vi "addNewMeasuredTemperature.vi"(8 "error in (no error)":errorcluster, 10 "Temperature Measured":dbl[unit]=275.15 min=271.15 max=275.15 format="%.1f", 11 "TestMonitor in":refnum<class "TestMonitor.lvclass">) -> (0 "error out":errorcluster, 3 "TestMonitor out":refnum<class "TestMonitor.lvclass">)   [LabVIEW 2013, in "TestMonitor.lvclass"]
uses:
  TestMonitor.lvclass
  TestMonitor.lvclass/TestMonitor.ctl
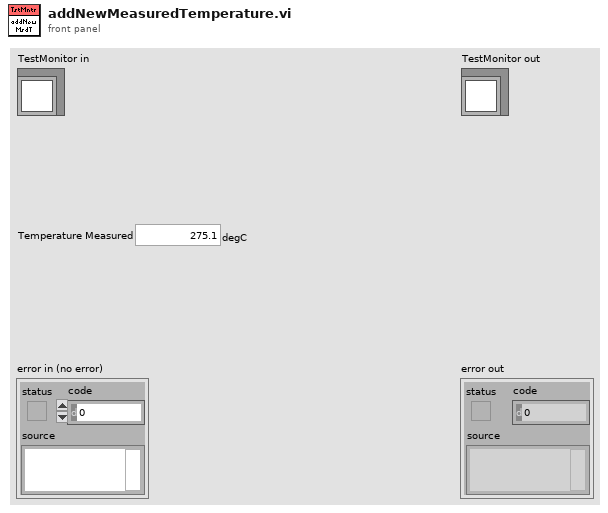
[diagram p1: front panel]
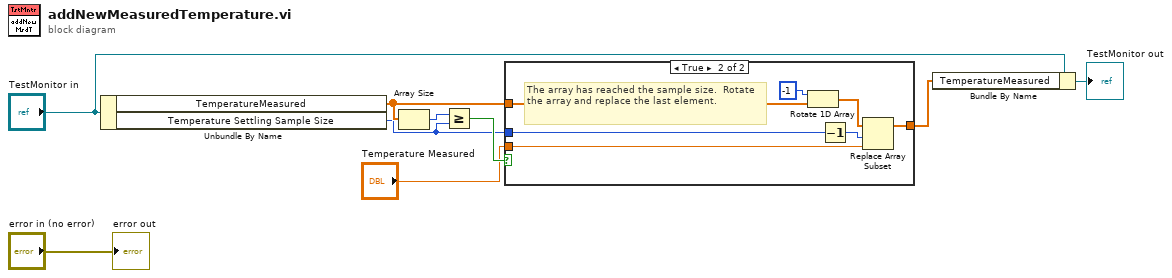
[diagram p0: block diagram]
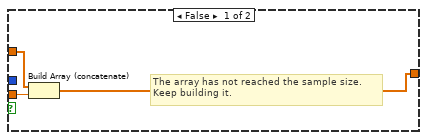
[diagram p2: hidden frame]
diagram:
  n1 = Unbundle By Name("TestMonitor in") -> ("TemperatureMeasured"=w4:dbl[unit][], "Temperature Settling Sample Size"=w1:u16)
  n2 = Array Size(array=w4) -> (size(s)=w6:i32)
  n3 = Greater Or Equal?(x=w6, y=w1) -> (x >= y?=w5:bool)
  n4 = case shown="True" w5 {
    tunnel: w4 -> [w12 w18]
    tunnel: "Temperature Measured" -> [w11 w14]
    tunnel: [w10 w13] -> w2
    tunnel: w1 -> [_ w15]
    frame False {
      # "The array has not reached the sample size.  Keep building it."
      n5 = Build Array (concatenate)(w12, w11) -> (w10:dbl[unit][])
    }
    frame True {
      # "The array has reached the sample size.  Rotate the array and replace the last element."
      n6 = Rotate 1D Array(1:w18, 2:-1 ("n")) -> (0:w19:dbl[unit][])
      n7 = Decrement(x=w15) -> (x-1=w16:u16)
      n8 = Replace Array Subset(array=w19, new element=w14, index=w16) -> (w13:dbl[unit][])
    }
  }
  n9 = Bundle By Name(cluster="TestMonitor in", "TemperatureMeasured"=w2) -> (→"TestMonitor out":refnum<class "TestMonitor.lvclass">)
  "error out" <- "error in (no error)"
